vi "StressDist_equivalent_VonMissesFormula.vi"(1 "Sshear":dbl, 2 "Scirc":dbl, 3 "Slong":dbl) -> (0 "Sequi":dbl)   [LabVIEW 2016]
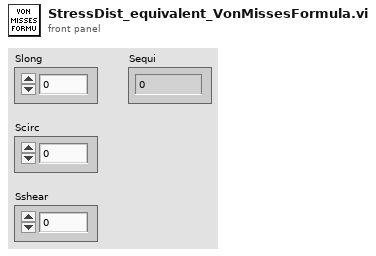
[diagram p1: front panel]
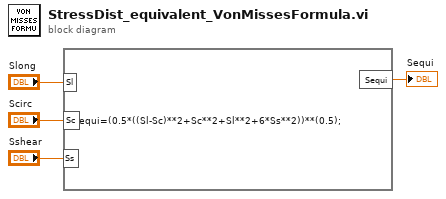
[diagram p0: block diagram]
diagram:
  n1 = formula code="Sequi=(0.5*((Sl-Sc)**2+Sc**2+Sl**2+6*Ss**2))**(0.5);"("Sl"="Slong", "Sc"="Scirc", "Ss"="Sshear") -> ("Sequi"=→"Sequi":dbl)
